vi "Create Pattern Script - Rd Capture Frame.vi"(8 "error in (no error)":errorcluster, 10 "FRM Data":T1 {"Addr" format="%x"; "Data" format="%x"}, 11 "SPI 4W Pattern Creator in":refnum<class "SPI 4W Pattern Creator.lvclass">) -> (0 "error out":errorcluster, 2 "String":string, 3 "SPI 4W Pattern Creator out":refnum<class "SPI 4W Pattern Creator.lvclass">)   [LabVIEW 2018, in "SPI 4W Pattern Creator.lvlib" / "SPI 4W Pattern Creator.lvclass"]
uses:
  SPI 4W Pattern Creator.lvclass
  Ctls/Frame Data - SPI_3W.ctl
  Ctls/RW Options.ctl
  Interfaces/Protocol Interface.lvlibp/Interfaces/Protocol Interface/Pin State.ctl
  Protocols/SPI Root Pattern Creator.lvlibp/Plugins/SouceCode/SPI_Pattern Creator/SPI Root/Data Type.ctl
  Protocols/SPI Root Pattern Creator.lvlibp/Plugins/SouceCode/SPI_Pattern Creator/SPI Root/Special Frame Type.ctl
  Interfaces/Protocol Interface.lvlibp/Interfaces/Protocol Interface/Protocol Interface.lvclass
  Protocols/SPI Root Pattern Creator.lvlibp/Plugins/SouceCode/SPI_Pattern Creator/SPI Root/SPI Root Pattern Creator.lvclass
  C:/P4 Workspace/PC Client/Solutions/5g_eap/trunk/1.0/HiSi5GmmWave/Pattern_Gen_Tool/Plugins/Protocols/SPI Root Pattern Creator.lvlibp/Plugins/SouceCode/SPI_Pattern Creator/SPI Root/SPI Root Pattern Creator.lvclass
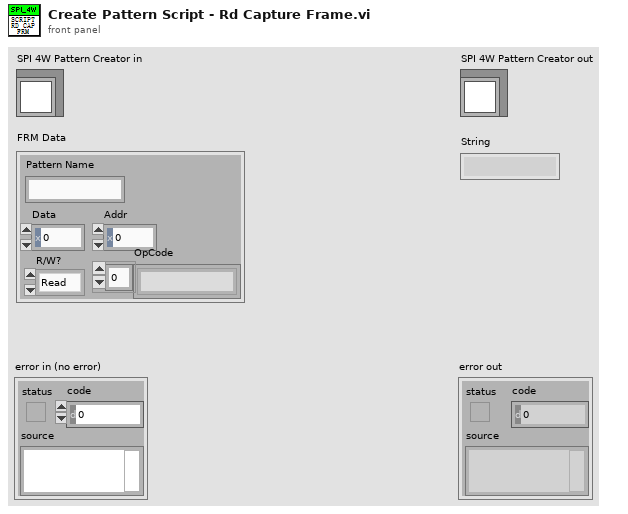
[diagram p1: front panel]
types:
  T1 = typedef "Frame Data - SPI_3W.ctl" = cluster{"Pattern Name":string, "Data":u16, "Addr":u16, "OpCode":string[], "R/W?":T2}
  T2 = typedef "RW Options.ctl" = enum16{"Read", "Write", "R/W"}
  T3 = typedef "SPI Root Pattern Creator.lvlibp/SPI Root Pattern Creator.lvclass/Special Frame Type.ctl" = enum16{"SPI 4W FRM Start", "SPI 4W Wait", "SPI 4W FRM End", "SPI 4W Write Cmd", "SPI Rd Collect Cmd", "SPI Rd Value Cmd", "SPI 3W FRM Start", "SPI 3W Write Cmd", "SPI 3W FRM End", "SPI 3W Wait", "SPI 3W Rd Cmd"}
  T4 = typedef "SPI Root Pattern Creator.lvlibp/SPI Root Pattern Creator.lvclass/Data Type.ctl" = enum16{"Drive", "Compare", "Read"}
  T5 = typedef "Protocol Interface.lvlibp/Protocol Interface.lvclass/Pin State.ctl" = enum16{"0", "1", "L", "H", "X", "V", "D", "M"}
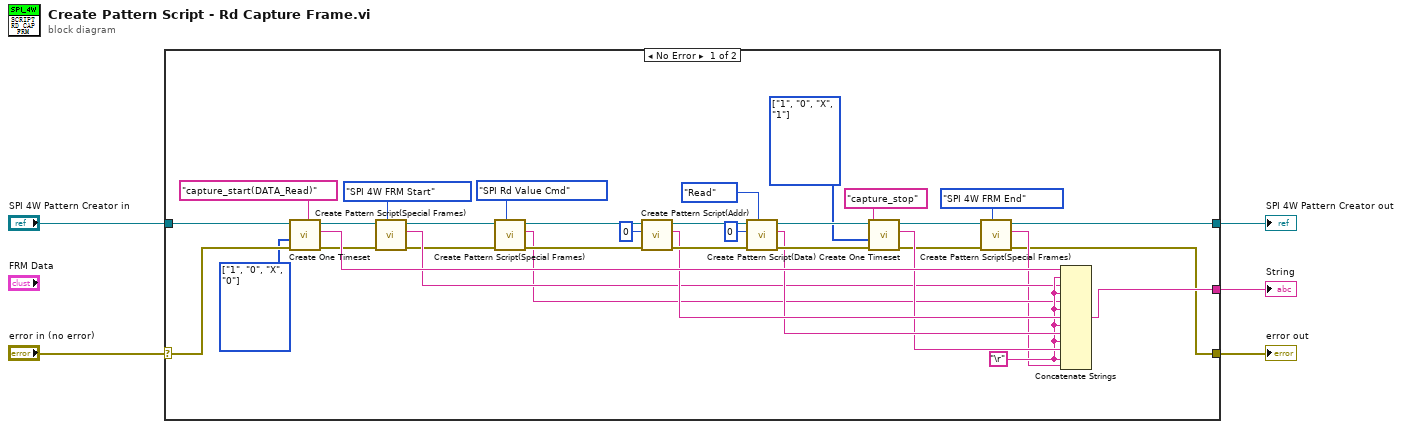
[diagram p0: block diagram]
diagram:
  n1 = case shown="No Error" "error in (no error)" {
    selector: "error in (no error)" -> [w36 w41]
    tunnel: "SPI 4W Pattern Creator in" -> [w37 w42]
    tunnel: [w10 w42] -> w2
    tunnel: [w9 w41] -> w1
    tunnel: [w23 _] -> w3
    frame No Error {
      w30 = T5[] [enum."1", enum."0", enum."X", enum."1"] items=["0", "1", "L", "H", "X", "V", "D", "M"] ("PinStates")
      w34 = T5[] [enum."1", enum."0", enum."X", enum."0"] items=["0", "1", "L", "H", "X", "V", "D", "M"] ("PinStates")
      w24 = "\r"
      n2 = call-dynamic "Create One Timeset.vi"("error in (no error)"=w36, "PinStates"=w34, "OpCode"="capture_start(DATA_Read)", "SPI 4W Pattern Creator in"=w37) -> ("error out"=w21:errorcluster, "String  out"=w28:string, "SPI 4W Pattern Creator out"=w22:refnum<class "SPI 4W Pattern Creator.lvclass">)  [unwired: 5 in]
      n3 = call "Create Pattern Script(Special Frames).vi"("Special Frame Type"=Special_Frame_Type."SPI 4W FRM Start", "error in (no error)"=w21, "SPI Root Pattern Creator in"=w22) -> ("error out"=w18:errorcluster, "String out"=w19:string, "SPI Root Pattern Creator out"=w20:refnum<class "SPI 4W Pattern Creator.lvclass">)  [unwired: 6 in]
      n4 = call "Create Pattern Script(Special Frames).vi"("Special Frame Type"=Special_Frame_Type."SPI Rd Value Cmd", "error in (no error)"=w18, "SPI Root Pattern Creator in"=w20) -> ("error out"=w17:errorcluster, "String out"=w15:string, "SPI Root Pattern Creator out"=w16:refnum<class "SPI 4W Pattern Creator.lvclass">)  [unwired: 6 in]
      n5 = call-dynamic "Create Pattern Script(Addr).vi"("error in (no error)"=w17, "Addr"=u16 0, "SPI 4W Pattern Creator in"=w16) -> ("error out"=w40:errorcluster, "String"=w27:string, "SPI 4W Pattern Creator out"=w39:refnum<class "SPI 4W Pattern Creator.lvclass">)  [unwired: 6 in]
      n6 = call-dynamic "Create Pattern Script(Data).vi"("Data Type"=Data_Type."Read", "error in (no error)"=w40, "Data"=u16 0, "SPI 4W Pattern Creator in"=w39) -> ("error out"=w31:errorcluster, "String"=w26:string, "SPI 4W Pattern Creator out"=w32:refnum<class "SPI 4W Pattern Creator.lvclass">)  [unwired: 5 in]
      n7 = call-dynamic "Create One Timeset.vi"("error in (no error)"=w31, "PinStates"=w30, "OpCode"="capture_stop", "SPI 4W Pattern Creator in"=w32) -> ("error out"=w12:errorcluster, "String  out"=w25:string, "SPI 4W Pattern Creator out"=w13:refnum<class "SPI 4W Pattern Creator.lvclass">)  [unwired: 5 in]
      n8 = call "Create Pattern Script(Special Frames).vi"("Special Frame Type"=Special_Frame_Type."SPI 4W FRM End", "error in (no error)"=w12, "SPI Root Pattern Creator in"=w13) -> ("error out"=w9:errorcluster, "String out"=w11:string, "SPI Root Pattern Creator out"=w10:refnum<class "SPI 4W Pattern Creator.lvclass">)  [unwired: 6 in]
      n9 = Concatenate Strings(w28, w24, w19, w24, w15, w24, w27, w24, w26, w24, w25, w24, w11) -> (w23:string)
    }
    frame Error {
    }
  }
  "error out" <- w1
  "SPI 4W Pattern Creator out" <- w2
  "String" <- w3
